vi "App_GetBuildInfoDevAndRunTime.vi"(8 "Error In":errorcluster) -> (0 "Error Out":errorcluster, 1 "FileVersionInfo Out":T1, 2 "FileVersion":string, 3 "InternalName":string)   [LabVIEW 2014]
uses:
  <vilib>/Platform/fileVersionInfo.llb/FileVersionInformation.ctl
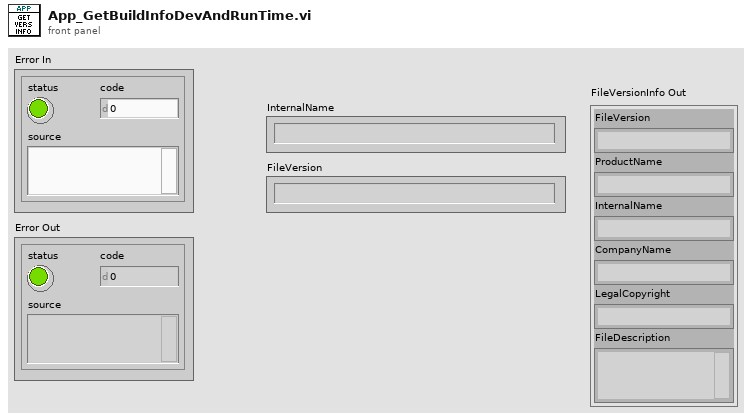
[diagram p1: front panel]
types:
  T1 = typedef "FileVersionInformation.ctl" = cluster{"FileVersion":string, "ProductName":string, "InternalName":string, "CompanyName":string, "LegalCopyright":string, "FileDescription":string}
  T2 = enum32{"invalid app kind", "Development System", "Run Time System", "Student Edition", "Embedded LabVIEW", "Evaluation", "Custom"}
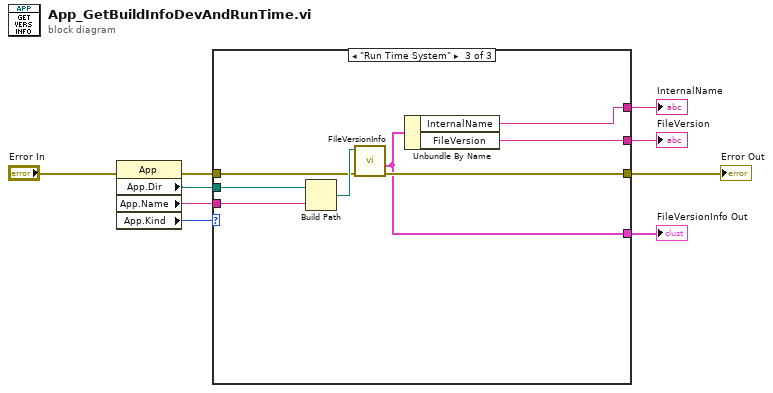
[diagram p0: block diagram]
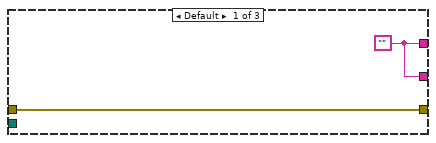
[diagram p2: hidden frame]
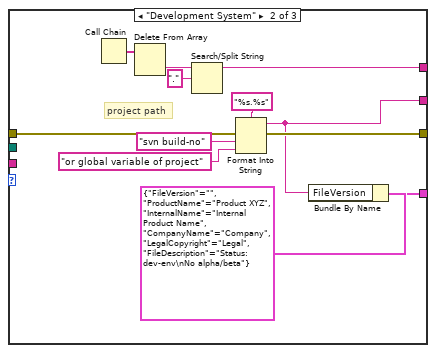
[diagram p3: hidden frame]
diagram:
  n1 = property class="App"(error in="Error In") -> (error out=w9:errorcluster, "App.Dir"=w8:path, "App.Name"=w7:string, "App.Kind"=w6:T2)  [unwired: 1 in, 1 out]
  n2 = case shown="\"Run Time System\"" w6 {
    tunnel: w9 -> [w11 w18 w30]
    tunnel: w8 -> [_ _ w29]
    tunnel: w7 -> [_ _ w28]
    tunnel: [w11 w22 w27] -> w3
    tunnel: [w10 w13 w26] -> w5
    tunnel: [w10 w12 w25] -> w4
    tunnel: [_ w14 w24] -> w1
    frame Default {
      w10 = ""
    }
    frame "Development System" {
      # "project path"
      n3 = Call Chain() -> (call chain=w23:string[])
      n4 = Delete From Array(array=w23) -> (deleted portion=w20:string)  [unwired: 2 in, 1 out]
      n5 = Search/Split String(string=w20, search string/char (-)=".") -> (substring before match=w13:string)  [unwired: 1 in, 2 out]
      n6 = Format Into String(format string="%s.%s", error in=w18, "svn build-no" ("input 1"), "or global variable of project" ("input 2")) -> (resulting string=w12:string, error out=w22:errorcluster)  [unwired: 1 in]
      n7 = Bundle By Name(cluster=T1 {"FileVersion"="", "ProductName"="Product XYZ", "InternalName"="Internal Product Name", "CompanyName"="Company", "LegalCopyright"="Legal", "FileDescription"="Status: dev-env\nNo alpha/beta"} ("FileVersionInfo Out"), "FileVersion"=w12) -> (w14:T1)
    }
    frame "Run Time System" {
      n8 = Build Path(base path=w29, name or relative path=w28) -> (appended path=w31:path)
      n9 = call <vilib>:"FileVersionInfo.vi"("error in (no error)"=w30, "Application Path in"=w31) -> ("error out"=w27:errorcluster, "FileVersionInfo Out"=w24:T1)  [unwired: 6 in, 2 out]
      n10 = Unbundle By Name(w24) -> ("InternalName"=w26:string, "FileVersion"=w25:string)
    }
  }
  "InternalName" <- w5
  "FileVersion" <- w4
  "Error Out" <- w3
  "FileVersionInfo Out" <- w1
